vi "Convert Image to JPG.vi"(8 "error in (no error)":errorcluster, 11 "Image Path in":path) -> (0 "error out":errorcluster, 3 "JPG Image Path out":path)   [LabVIEW 2015, in "Image Comparison.lvclass"]
uses:
  Image Comparison.lvclass
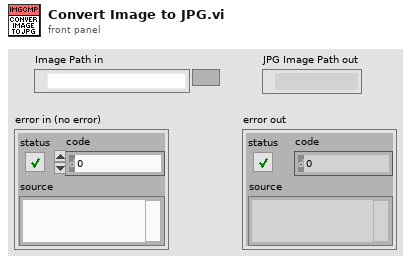
[diagram p1: front panel]
types:
  T1 = typedef "imagedata.ctl" = cluster{"image type":i32, "image depth":i32, "image":u8[], "mask":u8[], "colors":u32[], "Rectangle":cluster{"left":i16, "top":i16, "right":i16, "bottom":i16}}
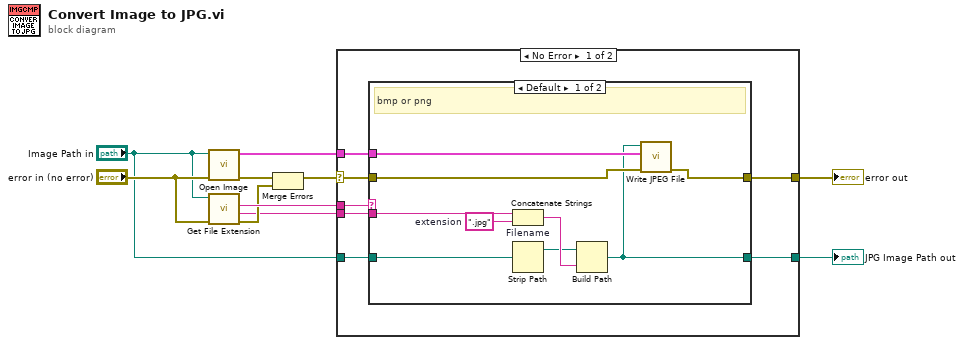
[diagram p0: block diagram]
diagram:
  n1 = call "Open Image.vi"("error in (no error)"="error in (no error)", "Image"="Image Path in") -> ("error out"=w8:errorcluster, "image data"=w5:T1)  [unwired: 8 in]
  n2 = call <vilib>:"Get File Extension.vi"("error in (no error)"="error in (no error)", "file"="Image Path in") -> ("error out"=w6:errorcluster, "filename without extension"=w4:string, "lowercase file extension"=w9:string)  [unwired: 5 in, 2 out]
  n3 = Merge Errors(w8, w6) -> (w7:errorcluster)
  n4 = case shown="No Error" w7 {
    selector: w7 -> [w16 w30]
    tunnel: w9 -> [w17 _]
    tunnel: w5 -> [w15 _]
    tunnel: w4 -> [w14 _]
    tunnel: [w13 w30] -> w3
    tunnel: [w12 w29] -> w2
    tunnel: "Image Path in" -> [w11 w29]
    frame No Error {
      n5 = case shown="Default" w17 {
        tunnel: w16 -> [w23 w28]
        tunnel: w15 -> [w24 _]
        tunnel: w14 -> [w26 _]
        tunnel: [w22 w28] -> w13
        tunnel: [w20 w27] -> w12
        tunnel: w11 -> [w19 w27]
        frame Default {
          w21 = ".jpg"  # extension
          # "bmp or png"
          n6 = Concatenate Strings "Filename"(w26, w21) -> (w25:string)
          n7 = Strip Path(path=w19) -> (stripped path=w18:path)  [unwired: 1 out]
          n8 = Build Path(base path=w18, name or relative path=w25) -> (appended path=w20:path)
          n9 = call <vilib>:"Write JPEG File.vi"("error in (no error)"=w23, "image data"=w24, "path to JPEG file"=w20) -> ("error out"=w22:errorcluster)  [unwired: 7 in, 1 out]
        }
        frame "jpg" {
          # "Already jpg"
        }
      }
    }
    frame Error {
    }
  }
  "error out" <- w3
  "JPG Image Path out" <- w2
